vi "GUI Monitoring Loop.vi"(8 "error in (no error)":errorcluster, 10 "Sync Objects":T1, 11 "FOFB Parameters":T2) -> (0 "error out":errorcluster)   [LabVIEW 2011, in "User Interface VIs.lvlib"]
uses:
  User Interface VIs.lvlib
  Types Definitions/Type FOFB Parameters.ctl
  Types Definitions/Type Network Configuration.ctl
  Types Definitions/Type FA Configuration.ctl
  Types Definitions/Type Response Matrix Measurement Configuration.ctl
  Types Definitions/Type Correction Algorithm Configuration.ctl
  Types Definitions/Type Acquisition Network Configuration.ctl
  Types Definitions/Type Actuation Network Configuration.ctl
  Types Definitions/Type FOFB GUI.ctl
  Types Definitions/Type Configuration Loop Mode.ctl
  Types Definitions/Type Configuration Data (GUI to Controller).ctl
  Types Definitions/Type Monitoring Data.ctl
  Types Definitions/Type Diagnostics Data.ctl
  Types Definitions/Type CPU Loads Array.ctl
  Types Definitions/Type CPU Loads.ctl
  Types Definitions/Type Diagnostics Sample.ctl
  Types Definitions/Type Monitoring Sample.ctl
  <vilib>/Platform/TimedLoop/XDataNode/timing_clust.ctl
  <vilib>/Platform/TimedLoop/XDataNode/nitl_modes.ctl
  <vilib>/Platform/TimedLoop/XDataNode/wakeup.ctl
  <vilib>/Platform/TimedLoop/XDataNode/XDataNode.xnode
  Type Definitions.lvlib
  <vilib>/Platform/TimedLoop/XDataNode/XDNodeRunTimeDep.lvlib
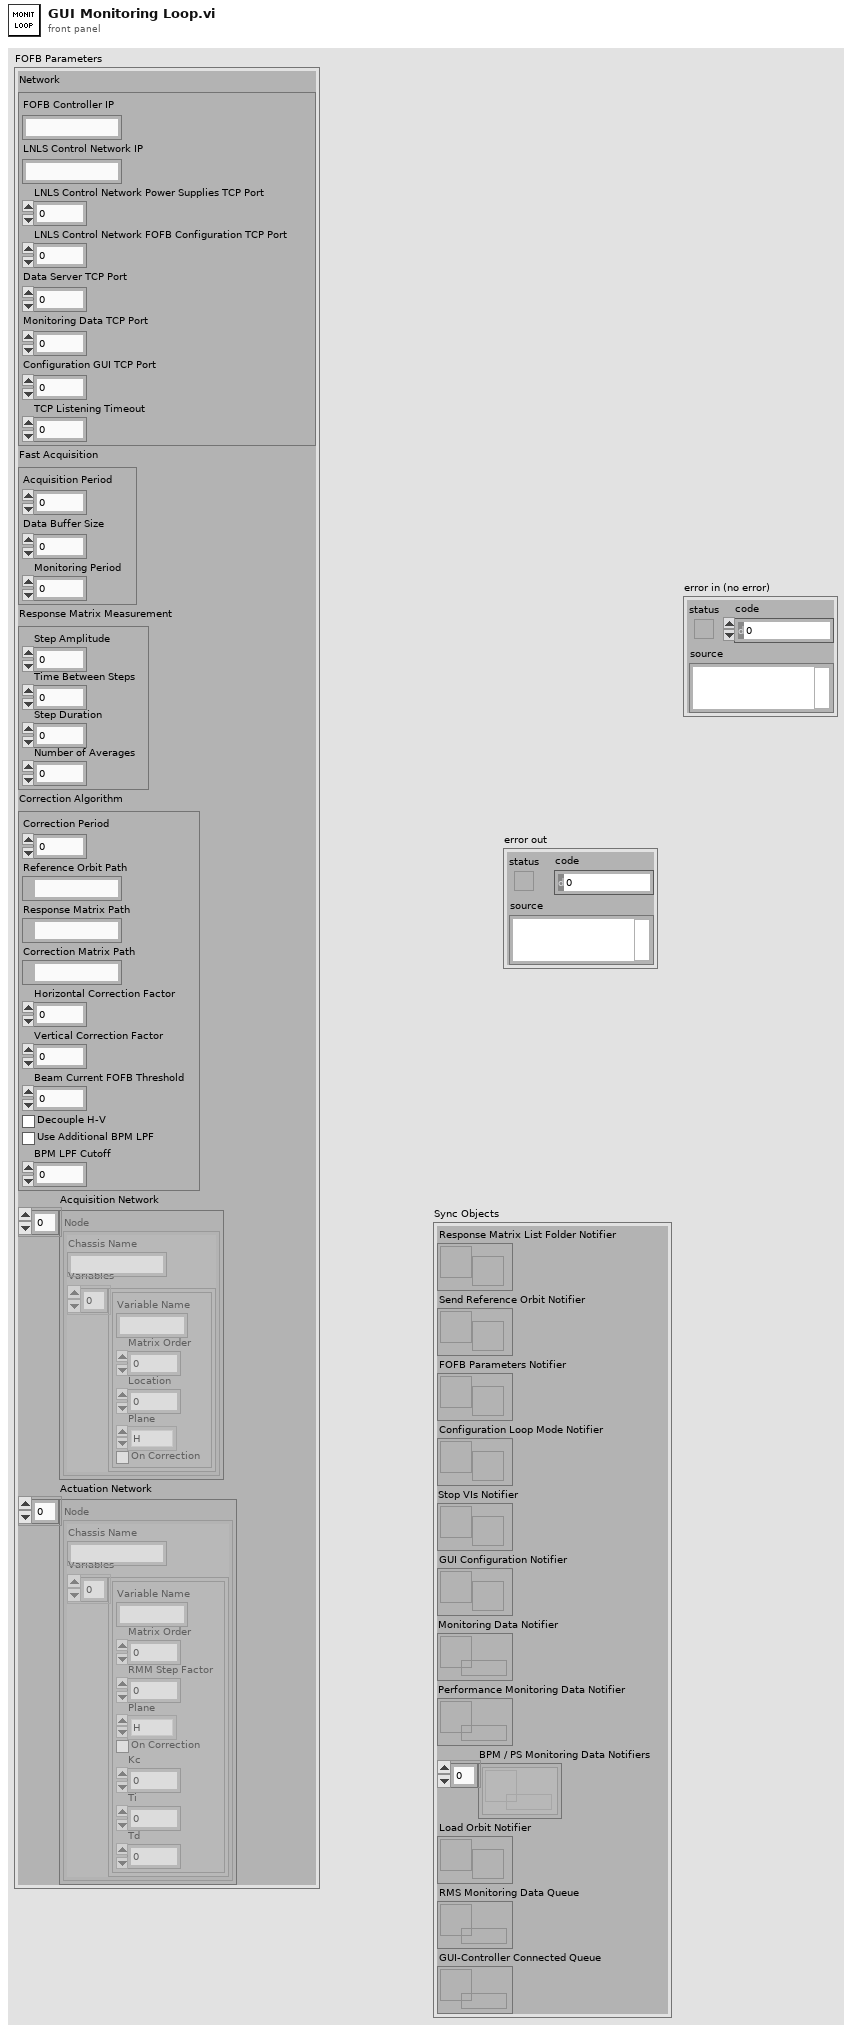
[diagram p1: front panel]
types:
  T1 = typedef "Type Definitions.lvlib/Type FOFB GUI.ctl" = cluster{"Response Matrix List Folder Notifier":refnum<notifier>, "Send Reference Orbit Notifier":refnum<notifier>, "FOFB Parameters Notifier":refnum<notifier>, "Configuration Loop Mode Notifier":refnum<notifier>, "Stop VIs Notifier":refnum<notifier>, "GUI Configuration Notifier":refnum<notifier>, "Monitoring Data Notifier":refnum<queue>, "Performance Monitoring Data Notifier":refnum<queue>, "BPM / PS Monitoring Data Notifiers":refnum<queue>[], "Load Orbit Notifier":refnum<notifier>, "RMS Monitoring Data Queue":refnum<queue>, "GUI-Controller Connected Queue":refnum<queue>}
  T2 = typedef "Type Definitions.lvlib/Type FOFB Parameters.ctl" = cluster{"Network":T3, "Fast Acquisition":T4, "Response Matrix Measurement":T5, "Correction Algorithm":T6, "Acquisition Network":T7, "Actuation Network":T8}
  T3 = typedef "Type Definitions.lvlib/Type Network Configuration.ctl" = cluster{"FOFB Controller IP":string, "LNLS Control Network IP":string, "LNLS Control Network Power Supplies TCP Port":u16, "LNLS Control Network FOFB Configuration TCP Port":u16, "Data Server TCP Port":u16, "Monitoring Data TCP Port":u16, "Configuration GUI TCP Port":u16, "TCP Listening Timeout":i32}
  T4 = typedef "Type Definitions.lvlib/Type FA Configuration.ctl" = cluster{"Acquisition Period":u32, "Data Buffer Size":u32, "Monitoring Period":u32}
  T5 = typedef "Type Definitions.lvlib/Type Response Matrix Measurement Configuration.ctl" = cluster{"Step Amplitude":dbl, "Time Between Steps":u32, "Step Duration":u32, "Number of Averages":u32}
  T6 = typedef "Type Definitions.lvlib/Type Correction Algorithm Configuration.ctl" = cluster{"Correction Period":u32, "Reference Orbit Path":path, "Response Matrix Path":path, "Correction Matrix Path":path, "Horizontal Correction Factor":dbl, "Vertical Correction Factor":dbl, "Beam Current FOFB Threshold":dbl, "Decouple H-V":bool, "Use Additional BPM LPF":bool, "BPM LPF Cutoff":dbl}
  T7 = typedef "Type Definitions.lvlib/Type Acquisition Network Configuration.ctl" = cluster{"Chassis Name":string, "Variables":cluster{"Variable Name":string, "Matrix Order":u32, "Location":dbl, "Plane":enum8{"H", "V"}, "On Correction":bool}[]}[]
  T8 = typedef "Type Definitions.lvlib/Type Actuation Network Configuration.ctl" = cluster{"Chassis Name":string, "Variables":cluster{"Variable Name":string, "Matrix Order":u32, "RMM Step Factor":dbl, "Plane":enum8{"H", "V"}, "On Correction":bool, "Kc":dbl, "Ti":dbl, "Td":dbl}[]}[]
  T9 = enum16{"Idle", "Wait Connection", "Read Data", "Close Connection"}
  T10 = typedef "XDNodeRunTimeDep.lvlib/timing_clust.ctl" = cluster{"Expected End [f-1]":u64, "Actual End [f-1]":u64, "Finished Late? [f-1]":bool, "Expected End [i-1]":u64, "Actual End [i-1]":u64, "Finished Late? [i-1]":bool, "Expected Start [i]":u64, "Actual Start [i]":u64, "Expected Start [f]":u64, "Actual Start [f]":u64, "Source Name":string, "Structure Name":string, "Period":i64, "Deadline":i64, "Offset":i64, "Start":i64, "Priority":i32, "Timeout":i32, "Mode":T11, "Wakeup Reason":T12, "Error":errorcluster, "Source Type":string, "Secondary Source Type":string, "Global End Time":u64, "Global Start Time":u64, "Frame Duration":u64, "Iteration Duration":u64, "Assigned CPU":i32, "I/O Scan Engine Mode":u32}
  T11 = typedef "XDNodeRunTimeDep.lvlib/nitl_modes.ctl" = enum32{"No Change", "Process missed periods, maintain original phase", "Discard missed periods, maintain original phase", "Process missed periods, ignore original phase", "Discard missed periods, ignore original phase"}
  T12 = typedef "XDNodeRunTimeDep.lvlib/wakeup.ctl" = enum32{"Normal", "Aborted", "Asynchronous wakeup", "Timing source error", "Timed loop error", "Timeout"}
  T13 = typedef "Type Definitions.lvlib/Type Monitoring Data.ctl" = cluster{"Timestamp":timestamp, "BPM Readings":dbl[], "PS Readings":dbl[], "PS FOFB Setpoints":dbl[], "PS Status per Rack":u8[], "PS ON-OFF per Rack":u8[], "Operation Mode":enum16{"Idle Mode", "Error Mode", "Manual Mode", "FOFB Mode", "RMM Mode"}, "Diagnostics Data":T14, "Controller Status Table":i32[]}
  T14 = typedef "Type Definitions.lvlib/Type Diagnostics Data.ctl" = cluster{"Time-Critical Loop Missed Iterations":u32, "Time-Critical Loop Execution Time (usec)":u32, "FA Buffer Usage":u32, "Available Memory (bytes)":u32, "CPU Loads Array":T15}
  T15 = typedef "Type Definitions.lvlib/Type CPU Loads Array.ctl" = T16[]
  T16 = typedef "Type Definitions.lvlib/Type CPU Loads.ctl" = cluster{"Total (%)":dbl, "Time Critical (%)":dbl, "Timed Structures (%)":dbl, "High (%)":dbl, "Above Normal (%)":dbl, "Normal (%)":dbl, "Background (%)":dbl, "Idle (%)":dbl, "ISR (%)":dbl}
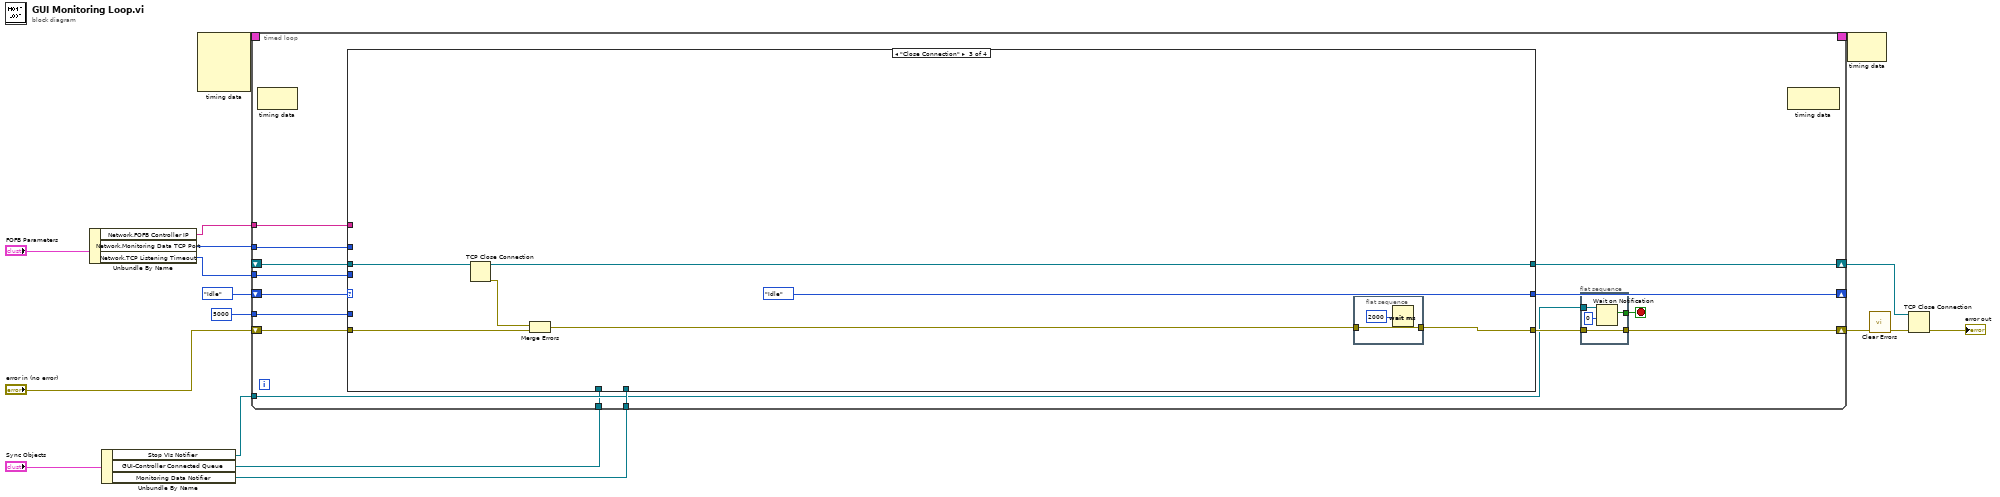
[diagram p0: block diagram]
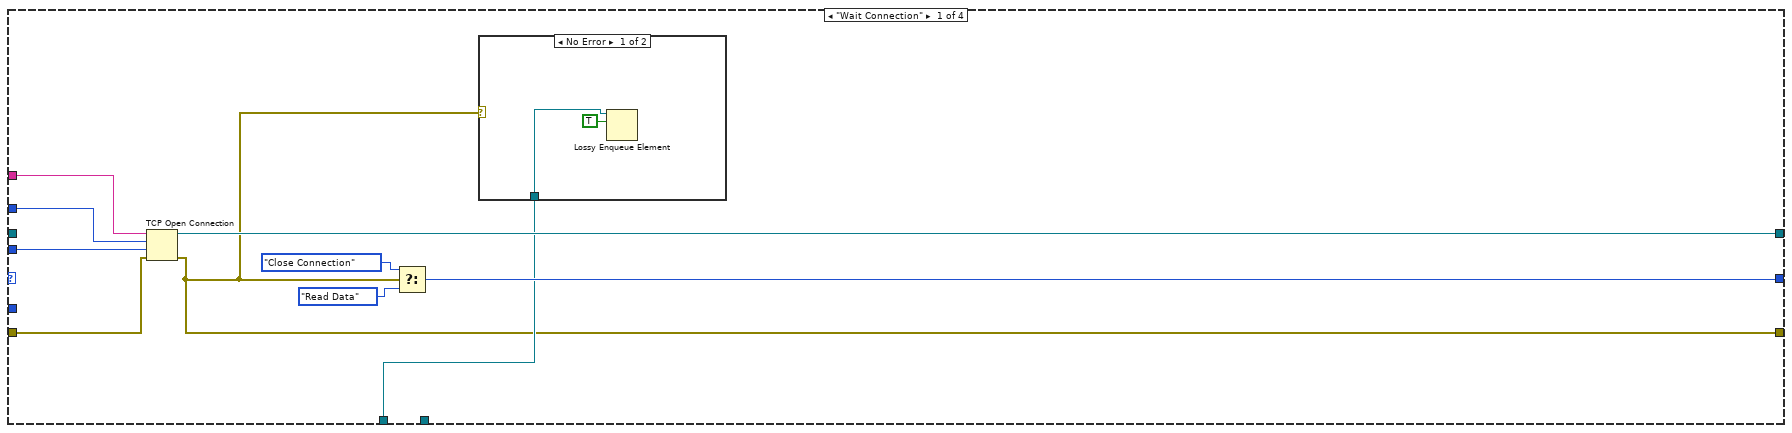
[diagram p2: hidden frame]
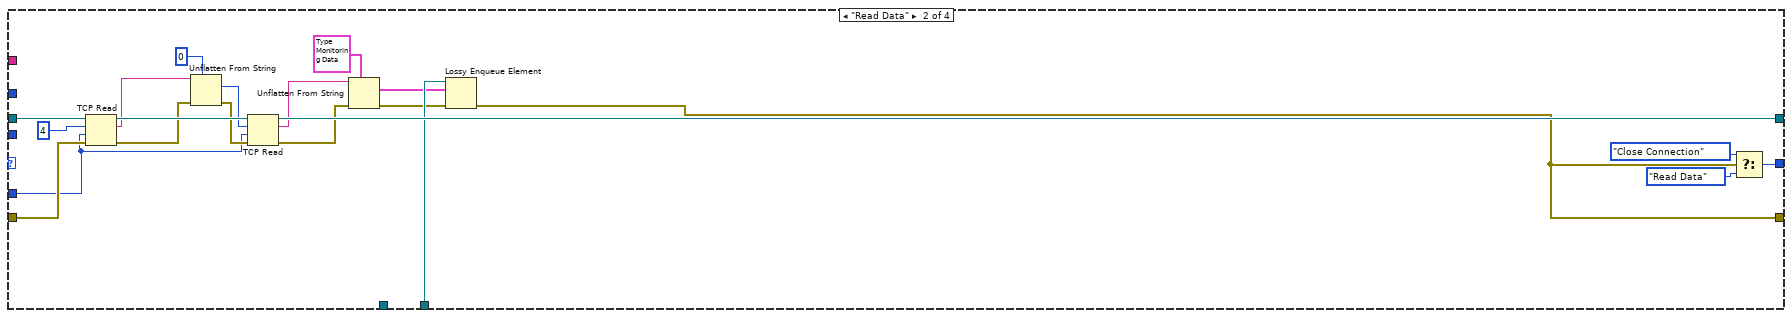
[diagram p4: hidden frame]
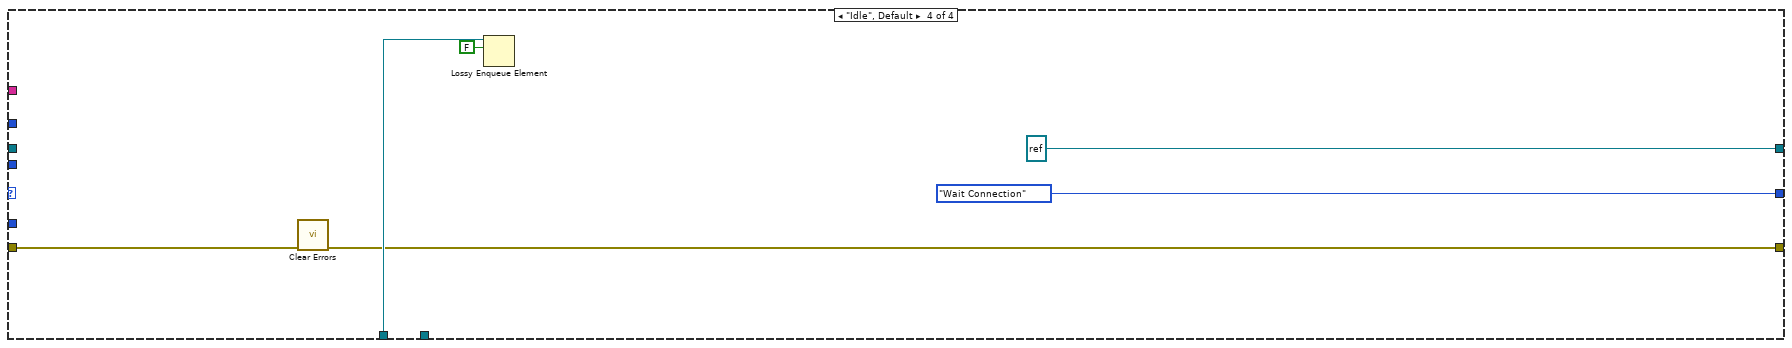
[diagram p5: hidden frame]
diagram:
  n1 = Unbundle By Name("FOFB Parameters") -> ("Network.FOFB Controller IP"=w2:string, "Network.Monitoring Data TCP Port"=w15:u16, "Network.TCP Listening Timeout"=w14:i32)
  n2 = Unbundle By Name("Sync Objects") -> ("Stop VIs Notifier"=w6:refnum<notifier>, "GUI-Controller Connected Queue"=w3:refnum<queue>, "Monitoring Data Notifier"=w5:refnum<queue>)
  n3 = node-c288() -> (w17:T10)  [unwired: 4 in]
  n4 = timed-loop {
    shift-right: [w23] -> w11
    shift-left: "error in (no error)" -> [w32]
    shift-right: [w28] -> _
    shift-left: T9."Idle" ("f") -> [w30]
    shift-right: [w29] -> w12
    shift-left: _ -> [w31]
    tunnel: w5 -> [w27]
    tunnel: w2 -> [w26]
    tunnel: w15 -> [w25]
    tunnel: w14 -> [w24]
    tunnel: w6 -> [w20]
    timing: w17 -> [_]
    timing-out: [_] -> w16
    tunnel: w3 -> [w19]
    tunnel: 5000 ("Network.TCP Listening Timeout") -> [w18]
    stop <- w21 stop-if-true
    n5 = node-c288() -> ()  [unwired: 1 in, 1 out]
    n6 = case shown="\"Close Connection\"" w30 {
      tunnel: [w48 w71 w78 refnum<k5> refnum ("connection ID")] -> w29
      tunnel: [w47 w70 T9."Idle" ("f") T9."Wait Connection" ("f")] -> w28
      tunnel: [w39 w52 w73 w81] -> w22
      tunnel: w32 -> [w46 w67 w74 w82]
      tunnel: w31 -> [_ w68 w77 _]
      tunnel: w27 -> [_ w58 _ _]
      tunnel: w26 -> [w43 _ _ _]
      tunnel: w25 -> [w42 _ _ _]
      tunnel: w24 -> [w41 _ _ _]
      tunnel: w19 -> [w40 _ _ w83]
      tunnel: w18 -> [_ w51 _ _]
      frame "Wait Connection" {
        n7 = TCP Open Connection(address=w43, remote port or service name=w42, timeout ms (60000)=w41, error in (no error)=w46) -> (connection ID=w48:refnum<k5>, error out=w39:errorcluster)  [unwired: 1 in]
        n8 = Select(t=T9."Close Connection" ("f"), s=w39, f=T9."Read Data") -> (s? t:f=w47:T9)
        n9 = case shown="No Error" w39 {
          tunnel: w40 -> [w49 _]
          frame No Error {
            n10 = Lossy Enqueue Element(queue=w49, element=TRUE ("notification")) -> ()  [unwired: 1 in, 4 out]
          }
          frame Error {
          }
        }
      }
      frame "Read Data" {
        n11 = TCP Read(connection ID=w68, bytes to read=4, error in (no error)=w67, 9:w51) -> (connection ID out=w69:refnum<k5>, data out=w63:string, error out=w53:errorcluster)  [unwired: 1 in]
        n12 = Unflatten From String(type=0 ("bytes to read"), binary string=w63, error in (no error)=w53) -> (value=w61:i32, error out=w57:errorcluster)  [unwired: 2 in, 1 out]
        n13 = TCP Read(connection ID=w69, bytes to read=w61, error in (no error)=w57, 9:w51) -> (connection ID out=w71:refnum<k5>, data out=w60:string, error out=w54:errorcluster)  [unwired: 1 in]
        n14 = Unflatten From String(type=T13 {"Timestamp"=timestamp(0 s since 1904-01-01), "BPM Readings"=[], "PS Readings"=[], "PS FOFB Setpoints"=[], "PS Status per Rack"=[], "PS ON-OFF per Rack"=[], "Operation Mode"=enum."Idle Mode", "Diagnostics Data"={"Time-Critical Loop Missed Iterations"=0, "Time-Critical Loop Execution Time (usec)"=0, "FA Buffer Usage"=0, "Available Memory (bytes)"=0, "CPU Loads Array"=[]}, "Controller Status Table"=[]} ("Slow Data"), binary string=w60, error in (no error)=w54) -> (value=w55:T13, error out=w56:errorcluster)  [unwired: 2 in, 1 out]
        n15 = Lossy Enqueue Element(queue=w58, element=w55, error in (no error)=w56) -> (error out=w52:errorcluster)  [unwired: 3 out]
        n16 = Select(t=T9."Close Connection" ("f"), s=w52, f=T9."Read Data") -> (s? t:f=w70:T9)
      }
      frame "Close Connection" {
        n17 = TCP Close Connection(connection ID=w77) -> (connection ID out=w78:refnum<k5>, error out=w75:errorcluster)  [unwired: 2 in]
        n18 = Merge Errors(w75, w74) -> (w72:errorcluster)
        n19 = flat-sequence {
          tunnel: [w80] -> w73
          tunnel: w72 -> [w80]
          frame #0 {
            n20 = Wait (ms)(milliseconds to wait=u32 2000 ("millisecond multiple")) -> ()  [unwired: 1 out]
          }
        }
      }
      frame "Idle", Default {
        n21 = call <vilib>:"Clear Errors.vi"("error in (no error)"=w82) -> ("error out"=w81:errorcluster)  [unwired: 6 in]
        n22 = Lossy Enqueue Element(queue=w83, element=FALSE ("notification")) -> ()  [unwired: 1 in, 4 out]
      }
    }
    n23 = flat-sequence {
      tunnel: [w38] -> w23
      tunnel: w22 -> [w38]
      tunnel: w20 -> [w37]
      tunnel: [w36] -> w21
      frame #0 {
        n24 = Wait on Notification(notifier=w37, timeout in ms (-1)=0) -> (notification=w36:bool)  [unwired: 2 in, 3 out]
      }
    }
    n25 = node-c288() -> ()  [unwired: 1 in, 1 out]
  }
  n26 = node-c288(w16) -> ()  [unwired: 1 out]
  n27 = call <vilib>:"Clear Errors.vi"("error in (no error)"=w11) -> ("error out"=w9:errorcluster)  [unwired: 6 in]
  n28 = TCP Close Connection(connection ID=w12, error in (no error)=w9) -> (error out=→"error out":errorcluster)  [unwired: 1 in, 1 out]
